vi "check Charge.vi"(8 "error in (no error)":errorcluster) -> (0 "error out":errorcluster)   [LabVIEW 2019]
uses:
  cmd_check charge.ctl
  _ctrl/init-r-stop.ctl
  _ctrl/system-status.ctl
  Glob_Ref.vi
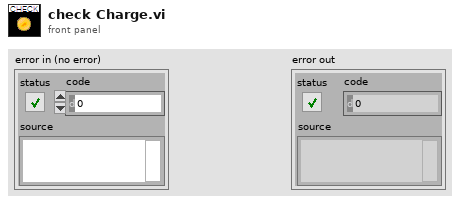
[diagram p1: front panel]
types:
  T1 = typedef "cmd_check charge.ctl" = enum16{"init", "run", "discharge", "disable", "close"}
  T2 = typedef "init-r-stop.ctl" = enum16{"ini", "read", "stop"}
  T3 = typedef "system-status.ctl" = enum16{"Initial", "Update", "Clear", "Read"}
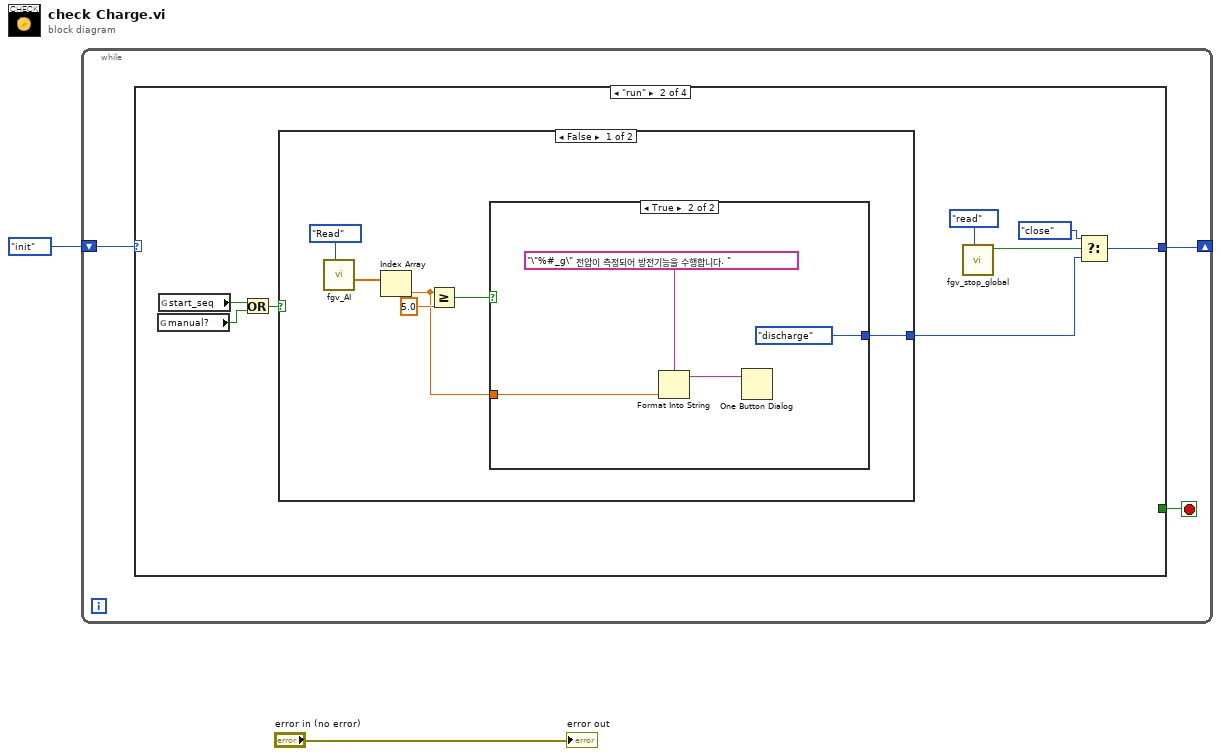
[diagram p0: block diagram]
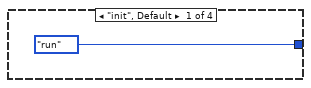
[diagram p2: hidden frame]
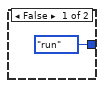
[diagram p3: hidden frame]
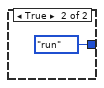
[diagram p4: hidden frame]
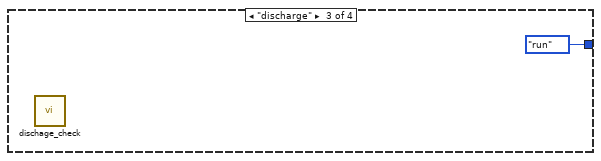
[diagram p5: hidden frame]
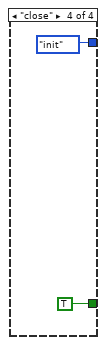
[diagram p6: hidden frame]
diagram:
  n1 = while {
    shift-right: [w4] -> _
    shift-left: cmd_check_charge."init" ("cmd") -> [w5]
    stop <- w3 stop-if-true
    n2 = case shown="\"run\"" w5 {
      tunnel: [cmd_check_charge."run" ("cmd") w11 cmd_check_charge."run" ("cmd") cmd_check_charge."init" ("cmd")] -> w4
      tunnel: [_ _ _ TRUE] -> w3
      frame "init", Default {
      }
      frame "run" {
        n3 = global read "Global_내구.vi" "manual?"() -> (w8:bool)
        n4 = global read "Glob_Ref.vi" "start_seq"() -> (w9:bool)
        n5 = Or(x=w9, y=w8) -> (x .or. y?=w7:bool)
        n6 = case shown="False" w7 {
          tunnel: [w15 cmd_check_charge."run" ("cmd")] -> w10
          frame False {
            n7 = call "fgv_AI.vi"("Mode"=system-status."Read") -> ("mean-vals"=w19:dbl[])  [unwired: 8 in, 2 out]
            n8 = Index Array(array=w19) -> (element=w16:dbl)  [unwired: 1 in]
            n9 = Greater Or Equal?(x=w16, y=5.0) -> (x >= y?=w17:bool)
            n10 = case shown="True" w17 {
              tunnel: w16 -> [_ w25]
              tunnel: [cmd_check_charge."run" ("cmd") cmd_check_charge."discharge" ("cmd")] -> w15
              frame False {
              }
              frame True {
                n11 = Format Into String(format string="\"%#_g\" 전압이 측정되어 방전기능을 수행합니다. ", w25) -> (resulting string=w23:string)  [unwired: 2 in, 1 out]
                n12 = One Button Dialog(message=w23) -> ()  [unwired: 1 in, 1 out]
              }
            }
          }
          frame True {
          }
        }
        n13 = call "fgv_stop_global.vi"("cmd"=init-r-stop."read") -> ("stop"=w13:bool)  [unwired: 10 in]
        n14 = Select(t=cmd_check_charge."close" ("cmd"), s=w13, f=w10) -> (s? t:f=w11:T1)
      }
      frame "discharge" {
        n15 = call "dischage_check.vi"() -> ()  [unwired: 11 in, 1 out]
      }
      frame "close" {
      }
    }
  }
  "error out" <- "error in (no error)"
